vi "Untitled 2.vi"() -> ()   [LabVIEW 2024]
uses:
  <vilib>/userDefined/High Color/IMAQdx.ctl
  <vilib>/vision/driver/NI_Vision_Acquisition_Software.lvlib
panel:
  in  "Senzor gaz":bool
  out "Senzor Gaz":bool
  out "Image":T1(plugin-control)
  in  "Session In":T2
  in  "stop":bool
  in  "stop 2":bool
  out "Senzor miscare   4":bool
  out "Senzor miscare   3":bool
  out "?":bool
  out "?":bool
  in  "Alarma miscare":bool
  out "Senzor miscare  5":bool
  out "Senzor miscare  4":bool
  out "Senzor miscare  3":bool
  out "Senzor miscare  2":bool
  out "Senzor miscare   2":bool
  out "Senzor miscare":bool
  out "?":bool
  out "?":bool
  out "?":bool
  out "?":bool
  out "?":bool
  out "?":bool
  out "?":bool
  out "?":bool
  out "?":bool
  out "?":bool
  out "?":bool
  in  "Temp.\nAfara":dbl(slide) scale=-30.0..40.0
  out "Degivrare \nNivel 1":bool
  out "Degivrare\nNivel 2":bool
  out "Dormitor I":bool
  out "Dormitor II":bool
  out "Sufragerie":bool
  out "Bucatarie":bool
  in  "Alarma incendiu":bool
  in  "Senzor Dormitor I":bool
  in  "Senzor Dormitor II":bool
  in  "Senzor Sufragerie":bool
  in  "Senzor Bucatarie":bool
  out "Comanda usi":string
  in  "Dormitor 1":bool
  in  "Bucatarie 2":bool
  in  "Sufragerie":bool
  in  "Bucatarie":bool
  in  "Bucatarie 2":bool
  in  "Debara 1":bool
  in  "Dormitor II":bool
  in  "Baie 2":bool
  in  "Baie 1":bool
  out "Usa baie 1":bool
  out "Usa baie 2":bool
  out "Usa dormitor II":bool
  out "Usa debara":bool
  out "Usa bucatarie 2":bool
  out "Usa bucatarie":bool
  out "Usa sufragerie":bool
  out "Usa dormitor":bool
  in  "Numeric 2":dbl
  in  "Numeric":dbl
  out "?":string
  out "Boolean 2":bool
  in  "Max 2":dbl
  in  "Min 2":dbl
  out "Temperatura":string
  in  "Temperatura":dbl(slide) scale=-20.0..60.0
  in  "Control umiditate":dbl(slide)=5.918367346938775 scale=0.0..10.0
  out "Atentie!\n Umiditate crescuta":bool
  out "Pornire ventilatie":bool
  out "Panou comanda usi":string
  out "?":string
  out "Usa birou":bool
  in  "Birou":bool
  in  "OK Button 2":bool
  out "?":string
  out "Usa intrare":bool
  in  "Intrare":bool
  in  "OK Button":bool
  out "Panou comanda geamuri":string
  in  "Geam Dormitor 1":bool
  in  "Geam Debara":bool
  in  "Geam Dormitor 2":bool
  in  "Geam Dormitor II":bool
  in  "Geam Birou":bool
  in  "Geam Bucatarie":bool
  in  "Geam Baie":bool
  in  "Geam Sufragerie":bool
  in  "Geam Hol":bool
  out "Geam Hol":bool
  out "Geam Dormitor II":bool
  out "Geam Baie'":bool
  out "Geam Dormitor 2":bool
  out "Geam Dormitor 1":bool
  out "Geam Sufragerie":bool
  out "Geam Bucatarie":bool
  out "Geam Debara":bool
  out "Geam Birou":bool
  # "Sistem Devrigare"
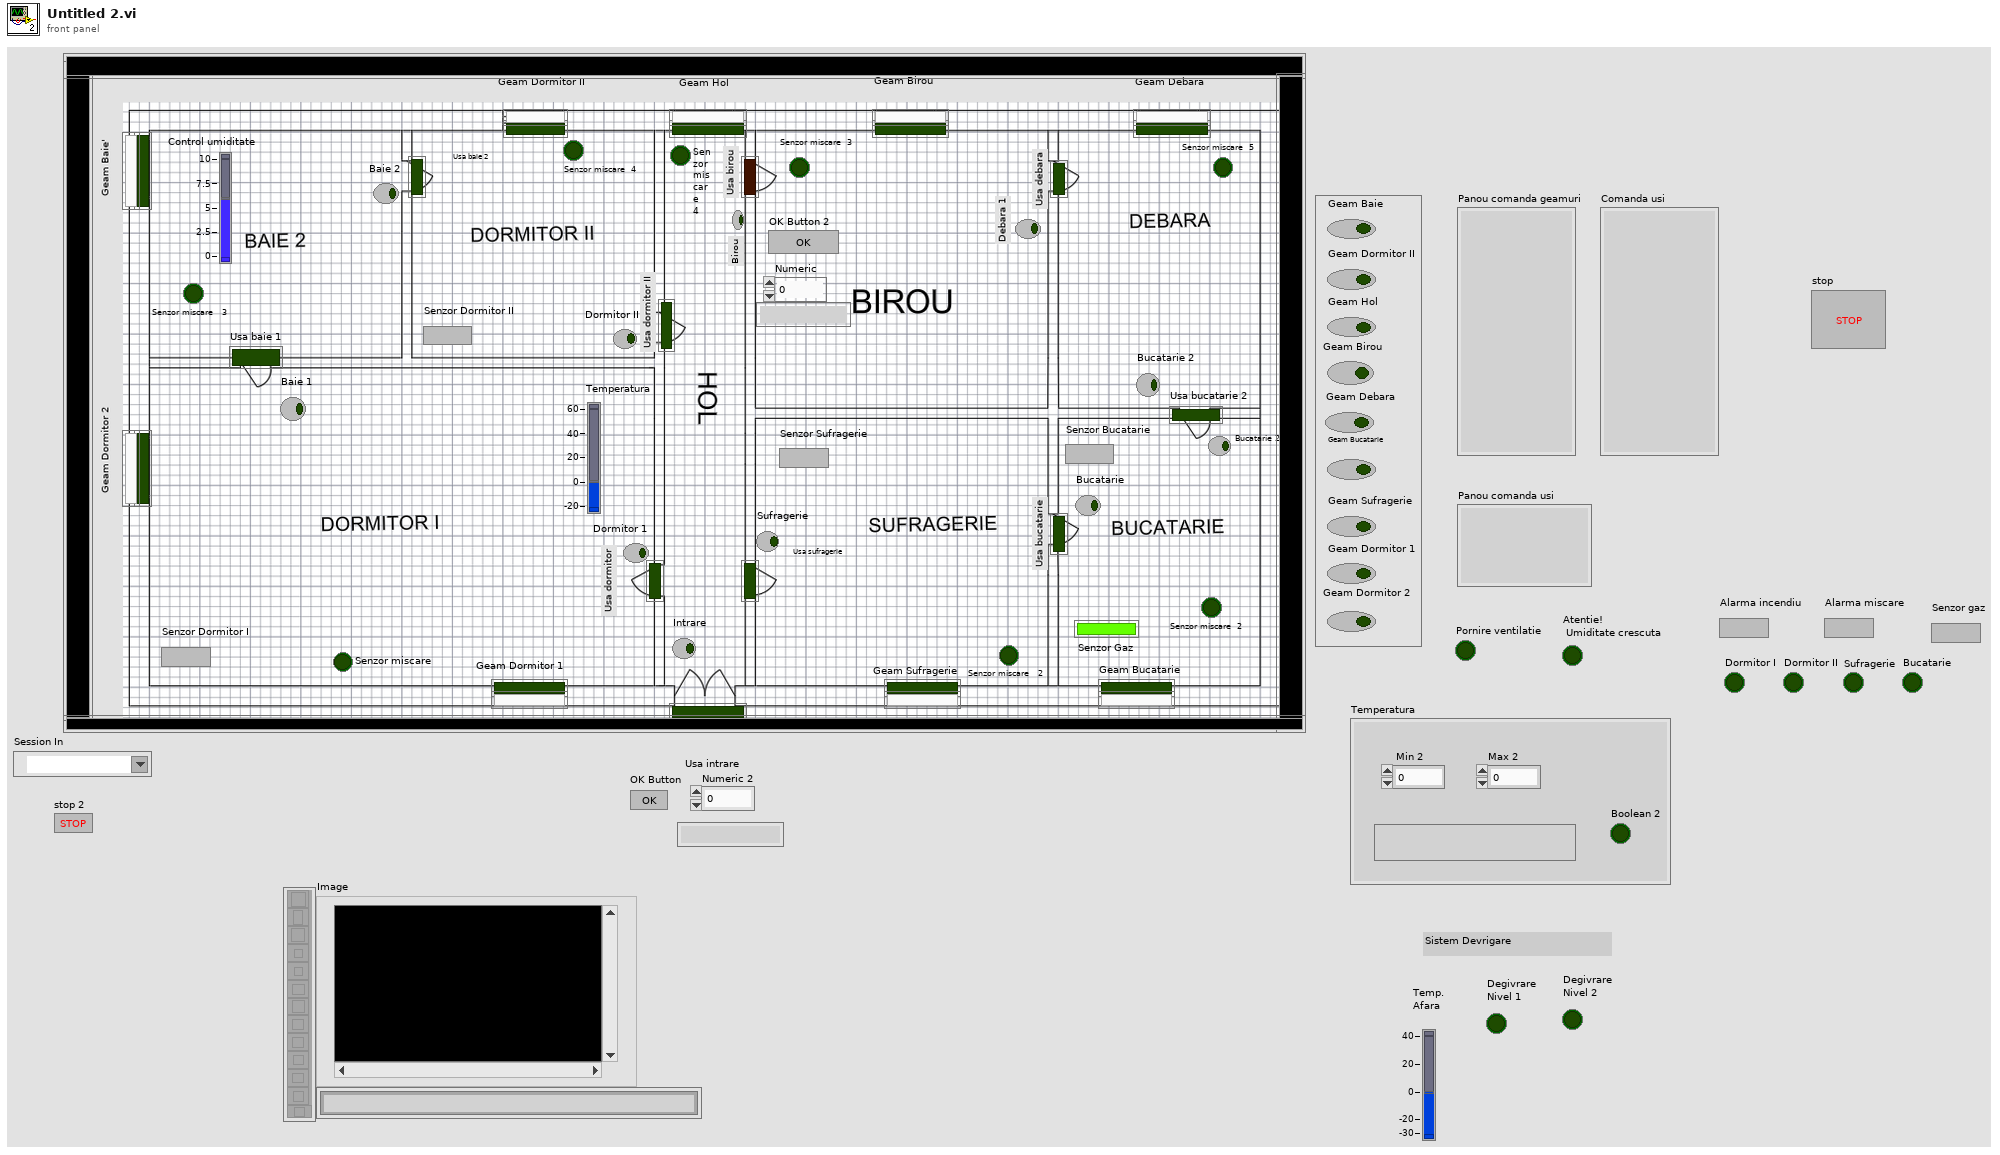
[diagram p1: front panel]
types:
  T1 = typedef "IMAQ Image.ctl" = refnum<image>
  T2 = typedef "IMAQdx.ctl" = refnum<k21>
  T3 = typedef "Image Type" = u32
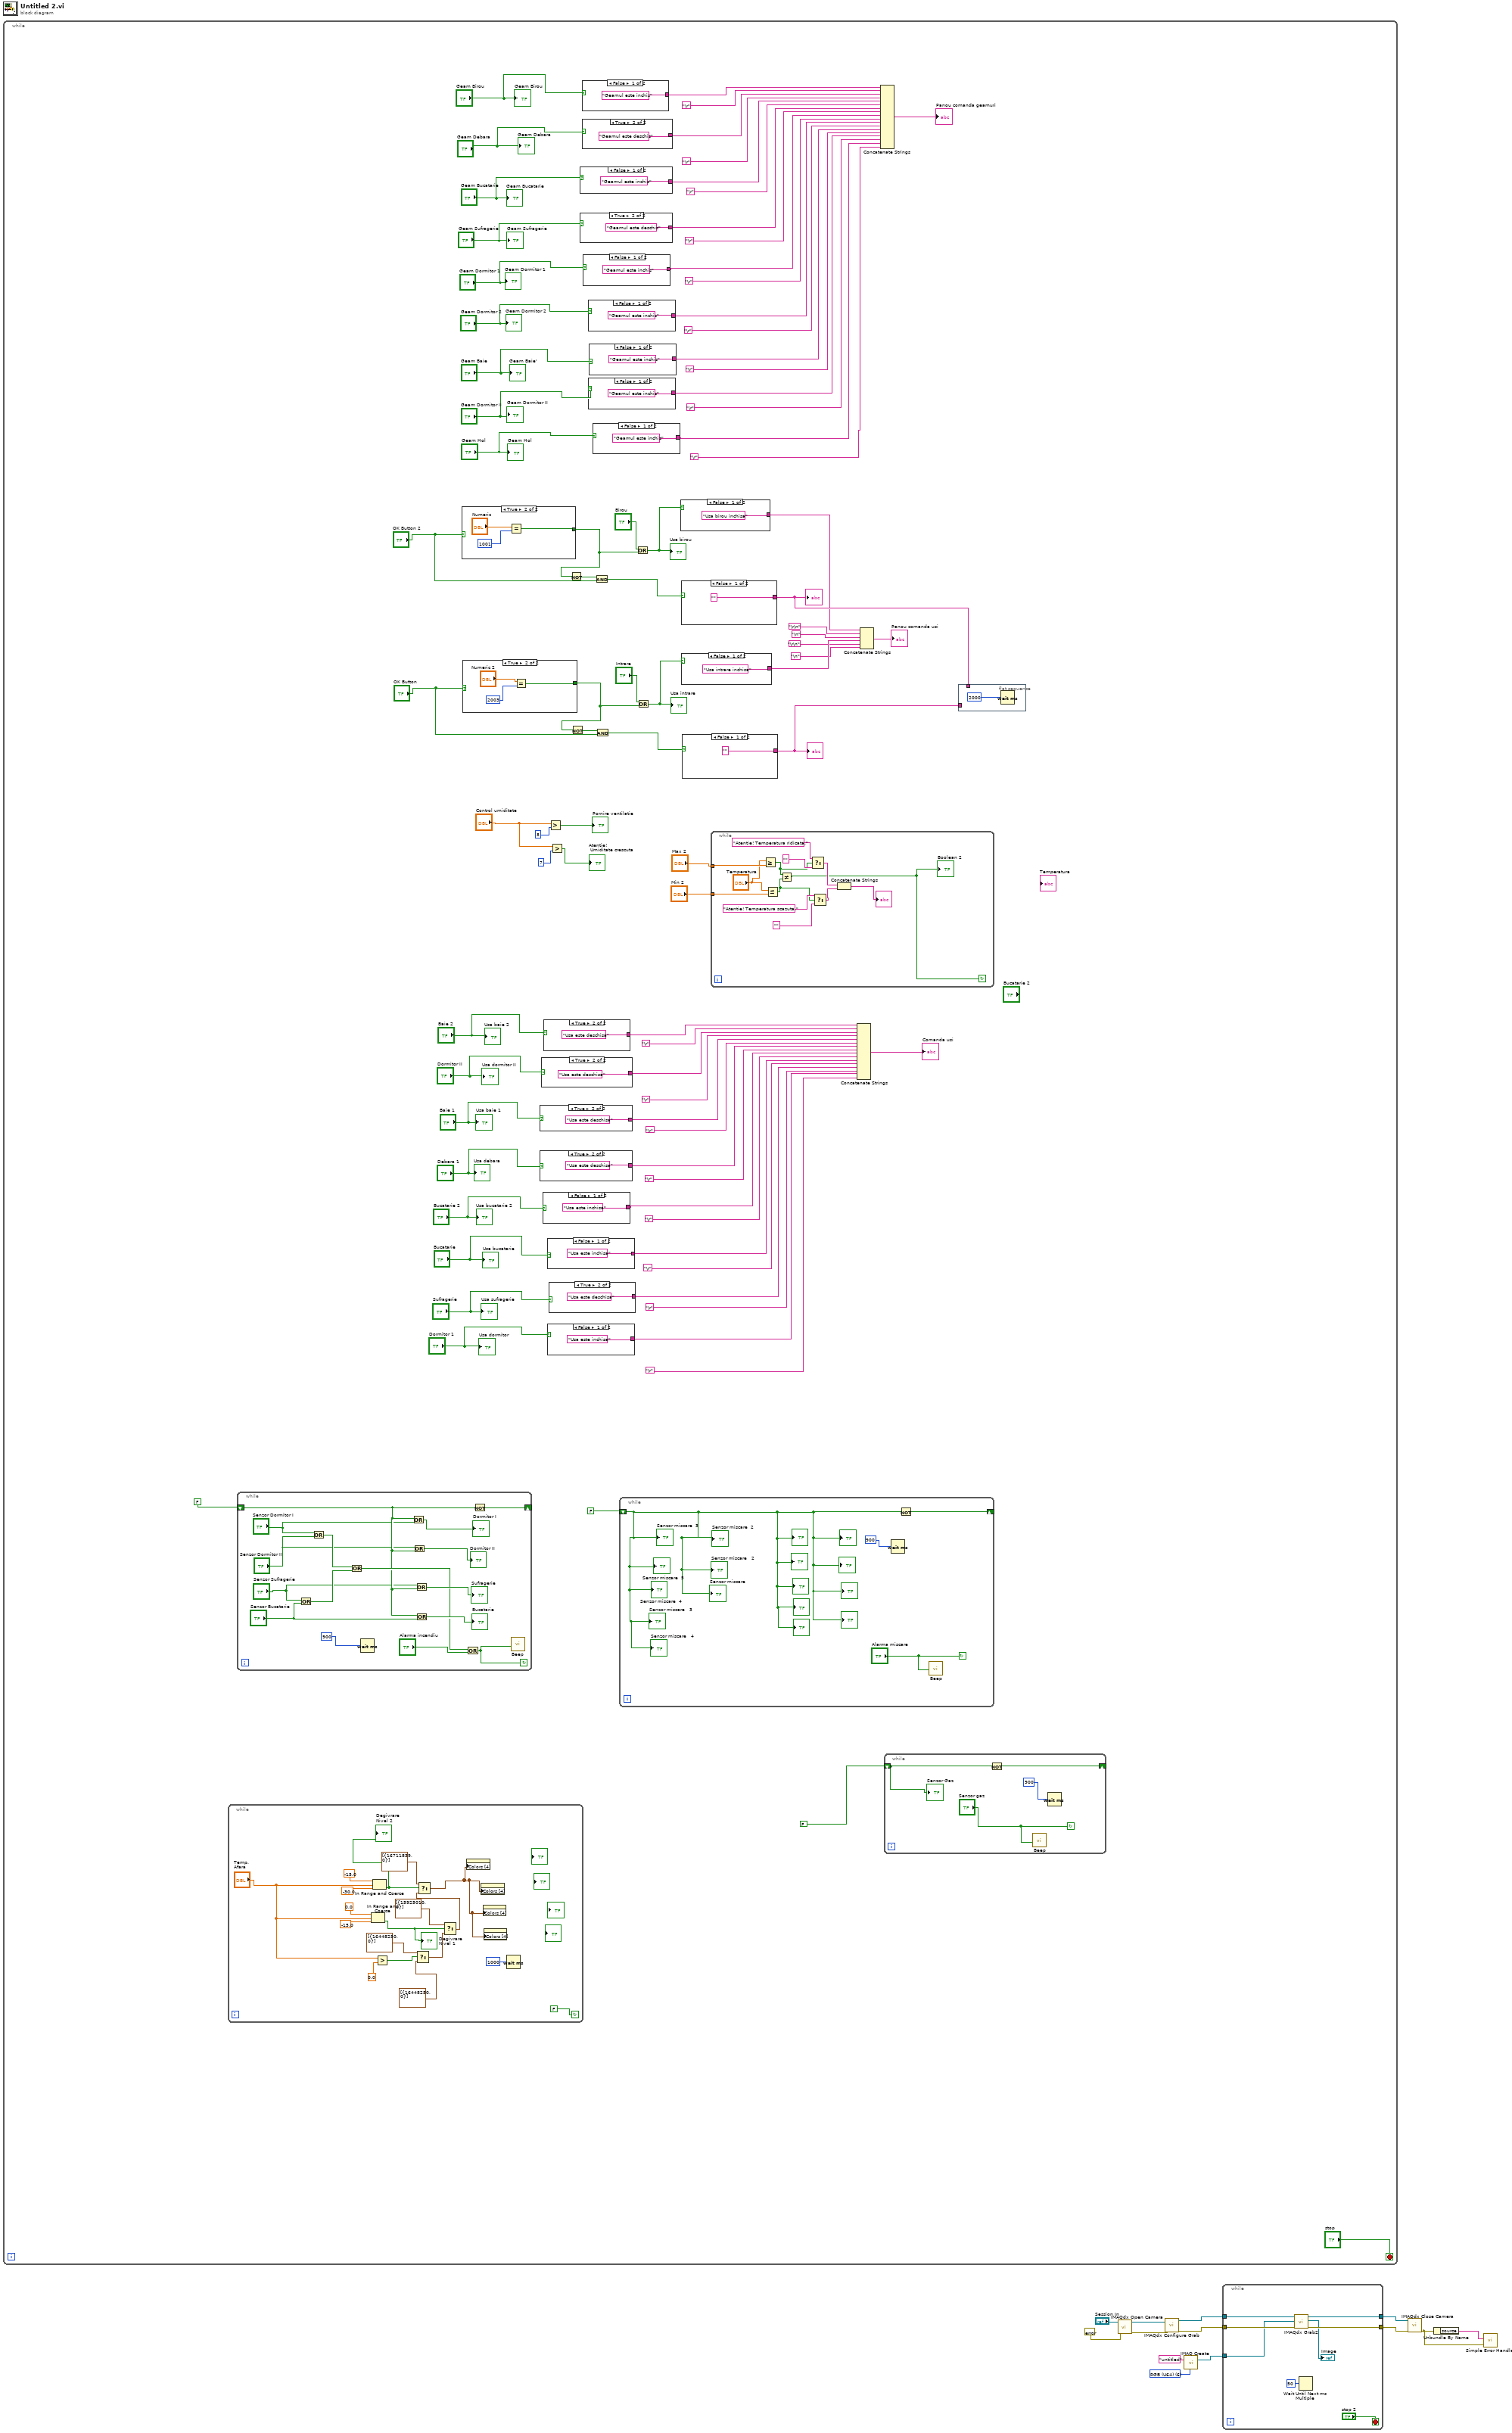
[diagram p0: block diagram]
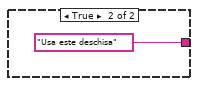
[diagram p2: hidden frame]
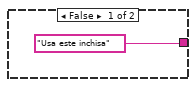
[diagram p3: hidden frame]
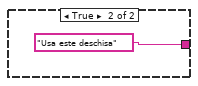
[diagram p4: hidden frame]
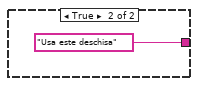
[diagram p5: hidden frame]
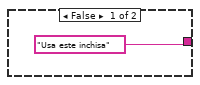
[diagram p6: hidden frame]
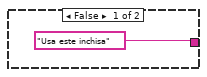
[diagram p7: hidden frame]
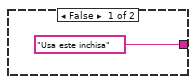
[diagram p8: hidden frame]
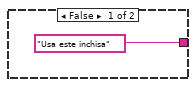
[diagram p9: hidden frame]
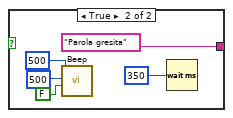
[diagram p10: hidden frame]
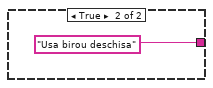
[diagram p11: hidden frame]
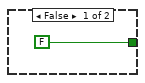
[diagram p12: hidden frame]
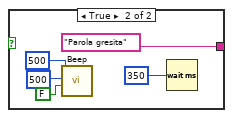
[diagram p13: hidden frame]
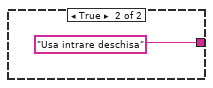
[diagram p14: hidden frame]
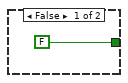
[diagram p15: hidden frame]
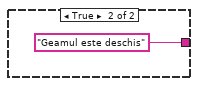
[diagram p16: hidden frame]
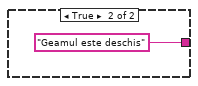
[diagram p17: hidden frame]
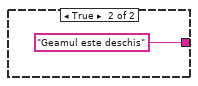
[diagram p18: hidden frame]
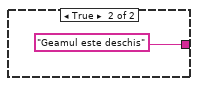
[diagram p19: hidden frame]
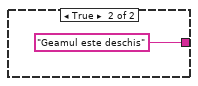
[diagram p20: hidden frame]
diagram:
  w4 = T3 6 items=["Grayscale (U8)", "Grayscale (I16)", "Grayscale (SGL)", "Complex (CSG)", "RGB (U32)", "HSL (U32)", "RGB (U64)", "Grayscale (U16)"] ("Image Type")
  n1 = while {
    stop <- "stop" stop-if-true
    n2 = while {
      stop <- FALSE continue-if-true
      n3 = In Range and Coerce(upper limit=0.0, x="Temp.\nAfara", lower limit=-15.0) -> (In Range?=w108:bool)  [unwired: 1 out]
      "Degivrare \nNivel 1" <- w108
      n4 = In Range and Coerce(upper limit=-15.0, x="Temp.\nAfara", lower limit=-30.0) -> (In Range?=w109:bool)  [unwired: 1 out]
      "Degivrare\nNivel 2" <- w109
      n5 = Greater?(x="Temp.\nAfara", y=0.0) -> (0:w115:bool)
      n6 = Select(t=cluster{u32, u32}[] [{16448250, 0}] ("Colors [4]"), s=w115, f=cluster{u32, u32}[] [{16448250, 0}] ("Colors [4]")) -> (s? t:f=w112:cluster{u32, u32}[])
      n7 = Select(t=cluster{u32, u32}[] [{15925010, 0}] ("Colors [4]"), s=w108, f=w112) -> (s? t:f=w117:cluster{u32, u32}[])
      n8 = Select(t=cluster{u32, u32}[] [{16711839, 0}] ("Colors [4]"), s=w109, f=w117) -> (s? t:f=w111:cluster{u32, u32}[])
      n9 = property class="Bool (strict)"("Colors [4]"=w111) -> ()  [unwired: 2 in, 2 out]
      n10 = property class="Bool (strict)"("Colors [4]"=w111) -> ()  [unwired: 2 in, 2 out]
      n11 = property class="Bool (strict)"("Colors [4]"=w111) -> ()  [unwired: 2 in, 2 out]
      n12 = property class="Bool (strict)"("Colors [4]"=w111) -> ()  [unwired: 2 in, 2 out]
      n13 = Wait (ms)(milliseconds to wait=u32 1000) -> ()  [unwired: 1 out]
    }
    n14 = while {
      shift-right: [w138] -> _
      shift-left: FALSE -> [w130]
      stop <- w132 continue-if-true
      n15 = Or(x="Senzor Sufragerie", y="Senzor Bucatarie") -> (x .or. y?=w139:bool)
      n16 = Or(x="Senzor Dormitor I", y="Senzor Dormitor II") -> (x .or. y?=w140:bool)
      n17 = Or(x=w140, y=w139) -> (x .or. y?=w133:bool)
      n18 = Wait (ms)(milliseconds to wait=900) -> ()  [unwired: 1 out]
      n19 = Or(x=w130, y="Senzor Dormitor I") -> (x .or. y?=→"Dormitor I":bool)
      n20 = Or(x="Senzor Dormitor II", y=w130) -> (x .or. y?=→"Dormitor II":bool)
      n21 = Or(x="Senzor Sufragerie", y=w130) -> (x .or. y?=→"Sufragerie":bool)
      n22 = Or(x=w130, y="Senzor Bucatarie") -> (x .or. y?=→"Bucatarie":bool)
      n23 = Or(x=w133, y="Alarma incendiu") -> (x .or. y?=w132:bool)
      n24 = Not(x=w130) -> (.not. x?=w138:bool)
      n25 = call <vilib>:"Beep.vi"("use system alert? (T)"=w132) -> ()  [unwired: 11 in]
    }
    n26 = case shown="True" "OK Button 2" {
      tunnel: [FALSE w181] -> w55
      frame False {
      }
      frame True {
        n27 = Equal?(x="Numeric", y=1001) -> (x = y?=w181:bool)
      }
    }
    n28 = case shown="True" "OK Button" {
      tunnel: [FALSE w194] -> w64
      frame False {
      }
      frame True {
        n29 = Equal?(x="Numeric 2", y=2003) -> (x = y?=w194:bool)
      }
    }
    n30 = case shown="True" "Baie 1" {
      tunnel: ["Usa este inchisa" "Usa este deschisa"] -> w31
      frame False {
      }
      frame True {
      }
    }
    n31 = case shown="True" "Debara 1" {
      tunnel: ["Usa este inchisa" "Usa este deschisa"] -> w33
      frame False {
      }
      frame True {
      }
    }
    n32 = case shown="True" "Dormitor II" {
      tunnel: ["Usa este inchisa" "Usa este deschisa"] -> w29
      frame False {
      }
      frame True {
      }
    }
    n33 = case shown="False" "Bucatarie 2" {
      tunnel: ["Usa este inchisa" "Usa este deschisa"] -> w35
      frame False {
      }
      frame True {
      }
    }
    n34 = case shown="True" "Baie 2" {
      tunnel: ["Usa este inchisa" "Usa este deschisa"] -> w27
      frame False {
      }
      frame True {
      }
    }
    n35 = case shown="False" "Dormitor 1" {
      tunnel: ["Usa este inchisa" "Usa este deschisa"] -> w41
      frame False {
      }
      frame True {
      }
    }
    n36 = case shown="False" "Bucatarie" {
      tunnel: ["Usa este inchisa" "Usa este deschisa"] -> w37
      frame False {
      }
      frame True {
      }
    }
    n37 = Greater?(x="Control umiditate", y=8) -> (0:→"Pornire ventilatie":bool)
    n38 = case shown="True" "Sufragerie" {
      tunnel: ["Usa este inchisa" "Usa este deschisa"] -> w39
      frame False {
      }
      frame True {
      }
    }
    n39 = Greater?(x="Control umiditate", y=7) -> (0:→"Atentie!\n Umiditate crescuta":bool)
    n40 = Not(x=w55) -> (.not. x?=w59:bool)
    n41 = Not(x=w64) -> (.not. x?=w69:bool)
    n42 = case shown="False" "Geam Bucatarie" {
      tunnel: ["Geamul este inchis" "Geamul este deschis"] -> w91
      frame False {
      }
      frame True {
      }
    }
    n43 = case shown="True" "Geam Sufragerie" {
      tunnel: ["Geamul este inchis" "Geamul este deschis"] -> w83
      frame False {
      }
      frame True {
      }
    }
    n44 = case shown="False" "Geam Birou" {
      tunnel: ["Geamul este inchis" "Geamul este deschis"] -> w97
      frame False {
      }
      frame True {
      }
    }
    n45 = case shown="True" "Geam Debara" {
      tunnel: ["Geamul este inchis" "Geamul este deschis"] -> w94
      frame False {
      }
      frame True {
      }
    }
    n46 = case shown="False" "Geam Dormitor 1" {
      tunnel: ["Geamul este inchis" "Geamul este deschis"] -> w81
      frame False {
      }
      frame True {
      }
    }
    n47 = case shown="False" "Geam Dormitor 2" {
      tunnel: ["Geamul este inchis" "Geamul este deschis"] -> w79
      frame False {
      }
      frame True {
      }
    }
    n48 = case shown="False" "Geam Dormitor II" {
      tunnel: ["Geamul este inchis" "Geamul este deschis"] -> w75
      frame False {
      }
      frame True {
      }
    }
    n49 = case shown="False" "Geam Baie" {
      tunnel: ["Geamul este inchis" "Geamul este deschis"] -> w77
      frame False {
      }
      frame True {
      }
    }
    n50 = case shown="False" "Geam Hol" {
      tunnel: ["Geamul este inchis" "Geamul este deschis"] -> w73
      frame False {
      }
      frame True {
      }
    }
    n51 = And(x=w59, y="OK Button 2") -> (x .and. y?=w57:bool)
    n52 = And(x=w69, y="OK Button") -> (x .and. y?=w66:bool)
    n53 = while {
      shift-right: [w105] -> _
      shift-left: FALSE -> [w103]
      stop <- "Alarma miscare" continue-if-true
      n54 = Wait (ms)(milliseconds to wait=900) -> ()  [unwired: 1 out]
      n55 = Not(x=w103) -> (.not. x?=w105:bool)
      n56 = call <vilib>:"Beep.vi"("use system alert? (T)"="Alarma miscare") -> ()  [unwired: 11 in]
      "Senzor miscare  5" <- w103
      "Senzor miscare  4" <- w103
      "Senzor miscare  3" <- w103
      "Senzor miscare  2" <- w103
      "Senzor miscare   2" <- w103
      "Senzor miscare" <- w103
      "?" <- w103
      "?" <- w103
      "?" <- w103
      "?" <- w103
      "?" <- w103
      "?" <- w103
      "?" <- w103
      "Senzor miscare   3" <- w103
      "Senzor miscare   4" <- w103
      "?" <- w103
      "?" <- w103
    }
    n57 = Or(x="Birou", y=w55) -> (x .or. y?=w60:bool)
    "Usa birou" <- w60
    n58 = Or(x="Intrare", y=w64) -> (x .or. y?=w70:bool)
    "Usa intrare" <- w70
    n59 = case shown="False" w60 {
      tunnel: ["Usa birou inchisa" "Usa birou deschisa"] -> w53
      frame False {
      }
      frame True {
      }
    }
    n60 = case shown="False" w57 {
      tunnel: ["" "Parola gresita"] -> w54
      frame False {
      }
      frame True {
        n61 = call <vilib>:"Beep.vi"("use system alert? (T)"=FALSE, "duration (msec)"=500, "frequency (Hz)"=500) -> ()  [unwired: 9 in]
        n62 = Wait (ms)(milliseconds to wait=350) -> ()  [unwired: 1 out]
      }
    }
    "?" <- w54
    n63 = case shown="False" w70 {
      tunnel: ["Usa intrare inchisa" "Usa intrare deschisa"] -> w63
      frame False {
      }
      frame True {
      }
    }
    n64 = case shown="False" w66 {
      tunnel: ["" "Parola gresita"] -> w67
      frame False {
      }
      frame True {
        n65 = call <vilib>:"Beep.vi"("use system alert? (T)"=FALSE, "duration (msec)"=500, "frequency (Hz)"=500) -> ()  [unwired: 9 in]
        n66 = Wait (ms)(milliseconds to wait=350) -> ()  [unwired: 1 out]
      }
    }
    "?" <- w67
    n67 = while {
      tunnel: "Max 2" -> [w164]
      tunnel: "Min 2" -> [w165]
      stop <- w157 continue-if-true
      n68 = Greater Or Equal?(x="Temperatura", y=w164) -> (x >= y?=w163:bool)
      n69 = Less Or Equal?(x="Temperatura", y=w165) -> (x <= y?=w162:bool)
      n70 = Not Equal?(x=w163, y=w162) -> (x != y?=w157:bool)
      "Boolean 2" <- w157
      n71 = Select(t="Atentie! Temperatura ridicata.", s=w163, f="") -> (s? t:f=w161:string)
      n72 = Select(t="Atentie! Temperatura scazuta.", s=w162, f="") -> (s? t:f=w160:string)
      n73 = Concatenate Strings(w161, w160) -> (→"?":string)
    }
    n74 = Concatenate Strings(w27, "\r", w29, "\r", w31, "\r", w33, "\r", w35, "\r", w37, "\r", w39, "\r", w41, "\r") -> (→"Comanda usi":string)
    n75 = Concatenate Strings(w53, "\r\n", "\n", w63, "\r\n", "\n") -> (→"Panou comanda usi":string)
    n76 = Concatenate Strings(w97, "\r", w94, "\r", w91, "\r", w83, "\r", w81, "\r", w79, "\r", w77, "\r", w75, "\r", w73, "\r") -> (→"Panou comanda geamuri":string)
    n77 = while {
      shift-right: [w102] -> _
      shift-left: FALSE -> [w100]
      stop <- "Senzor gaz" continue-if-true
      n78 = Not(x=w100) -> (.not. x?=w102:bool)
      n79 = call <vilib>:"Beep.vi"("use system alert? (T)"="Senzor gaz") -> ()  [unwired: 11 in]
      n80 = Wait (ms)(milliseconds to wait=900) -> ()  [unwired: 1 out]
      "Senzor Gaz" <- w100
    }
    n81 = flat-sequence {
      tunnel: w67 -> [_]
      tunnel: w54 -> [_]
      frame #0 {
        n82 = Wait (ms)(milliseconds to wait=2000) -> ()  [unwired: 1 out]
      }
    }
    "Geam Birou" <- "Geam Birou"
    "Geam Debara" <- "Geam Debara"
    "Geam Bucatarie" <- "Geam Bucatarie"
    "Geam Sufragerie" <- "Geam Sufragerie"
    "Geam Dormitor 1" <- "Geam Dormitor 1"
    "Geam Dormitor 2" <- "Geam Dormitor 2"
    "Geam Baie'" <- "Geam Baie"
    "Geam Dormitor II" <- "Geam Dormitor II"
    "Geam Hol" <- "Geam Hol"
    "Usa dormitor" <- "Dormitor 1"
    "Usa sufragerie" <- "Sufragerie"
    "Usa bucatarie" <- "Bucatarie"
    "Usa bucatarie 2" <- "Bucatarie 2"
    "Usa debara" <- "Debara 1"
    "Usa dormitor II" <- "Dormitor II"
    "Usa baie 2" <- "Baie 2"
    "Usa baie 1" <- "Baie 1"
  }
  n83 = call <vilib>:"IMAQdx Open Camera.vi"("error in"=errorcluster {"status"=FALSE, "code"=0, "source"=""}, "Session In"="Session In") -> ("error out"=w9:errorcluster, "Session Out"=w11:T2)  [unwired: 8 in]
  n84 = call <vilib>:"IMAQdx Configure Grab.vi"("error in"=w9, "Session In"=w11) -> ("error out"=w8:errorcluster, "Session Out"=w10:T2)  [unwired: 8 in]
  n85 = call "IMAQ Create"("Image Name"="untitled", "Image Type"=w4) -> ("New Image"=w3:T1)  [unwired: 3 in, 1 out]
  n86 = while {
    tunnel: w10 -> [w219]
    tunnel: w8 -> [w218]
    tunnel: [w217] -> w7
    tunnel: [w216] -> w6
    tunnel: w3 -> [w215]
    stop <- "stop 2" stop-if-true
    n87 = call <vilib>:"IMAQdx Grab2.vi"("error in"=w218, "Image In"=w215, "Session In"=w219) -> ("error out"=w216:errorcluster, "Image Out"=→"Image":T1, "Session Out"=w217:T2)  [unwired: 5 in, 1 out]
    n88 = Wait Until Next ms Multiple(millisecond multiple=u32 50) -> ()  [unwired: 1 out]
  }
  n89 = call <vilib>:"IMAQdx Close Camera.vi"("error in"=w6, "Session In"=w7) -> ("error out"=w2:errorcluster)  [unwired: 9 in]
  n90 = Unbundle By Name(w2) -> ("source"=w1:string)
  n91 = call <vilib>:"Simple Error Handler.vi"("error source (\" \")"=w1, "error in (no error)"=w2) -> ()  [unwired: 3 in, 5 out]
